vi "Multify(I64[]).vi"(1 "启用（T）":bool=TRUE, 2 "In":i64[](array[numeric]), 4 "n":i64=1) -> (6 "Out":i64[](array[numeric]))   [LabVIEW 2011]
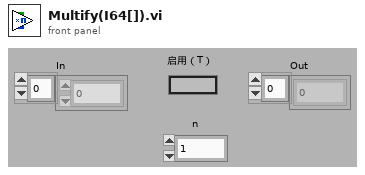
[diagram p1: front panel]
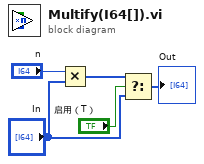
[diagram p0: block diagram]
diagram:
  n1 = Multiply(x="n", y="In") -> (x*y=w1:i64[])
  n2 = Select(t=w1, s="启用（T）", f="In") -> (s? t:f=→"Out":i64[])
